vi "_Request Malloc Memory To Factory.vi"(10 "error in (no error)":errorcluster, 11 "CacheSize":i32) -> (2 "error out":errorcluster, 3 "MDPtr DVR":refnum<data-value>)   [LabVIEW 2017, in "MDPtr.lvlib" / "MDPtrMgr.lvclass"]
uses:
  MDPtrMgr.lvclass
  MDPtr TypeDef/MDPtr DataFrame-Memory.ctl
  MDPtr TypeDef/MDPtr DataFrame-Common.ctl
  <vilib>/Utility/Data Type/Type Definitions/Data Type.ctl
  Def-Request.ctl
  Def-Respone.ctl
  MDPtr TypeDef/MDPtr Queue.ctl
  <vilib>/Utility/Data Type/NI_Data Type.lvlib
  MDPtr.lvlib
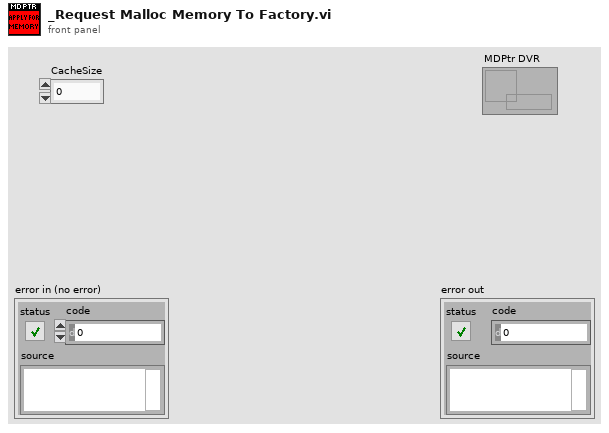
[diagram p1: front panel]
types:
  T1 = typedef "MDPtr.lvlib/MDPtrMgr.lvclass/Def-Respone.ctl" = cluster{"MDPtr DVR":refnum<data-value>, "error out":errorcluster, "MDPtrQueue":T2}
  T2 = typedef "MDPtr.lvlib/MDPtr Queue.ctl" = refnum<queue>
  T3 = typedef "MDPtr.lvlib/MDPtrMgr.lvclass/Def-Request.ctl" = cluster{"Type":enum16{"DVR", "Queue"}, "Cache Length":i32, "ResponeQueue":refnum<queue>}
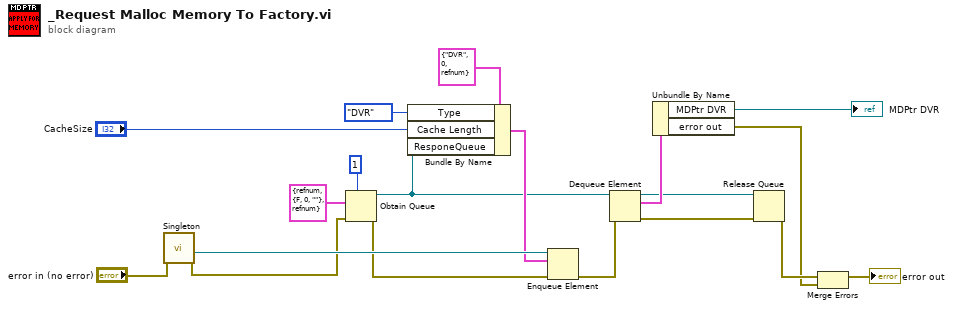
[diagram p0: block diagram]
diagram:
  n1 = call "Singleton.vi"("error in (no error)"="error in (no error)") -> ("error out"=w1:errorcluster, "RequestQueue"=w19:refnum<queue>)  [unwired: 8 in, 1 out]
  n2 = Obtain Queue(max queue size (-1, unlimited)=1, element data type=T1 {"MDPtr DVR"=refnum, "error out"={"status"=FALSE, "code"=0, "source"=""}, "MDPtrQueue"=refnum} ("Request"), error in (no error)=w1) -> (queue out=w11:refnum<queue>, error out=w13:errorcluster)  [unwired: 2 in, 1 out]
  n3 = Bundle By Name(cluster=T3 {"Type"=enum."DVR", "Cache Length"=0, "ResponeQueue"=refnum} ("element"), "Type"=enum16{"DVR", "Queue"}."DVR", "Cache Length"="CacheSize", "ResponeQueue"=w11) -> (w17:T3)
  n4 = Enqueue Element(queue=w19, element=w17, error in (no error)=w13) -> (error out=w10:errorcluster)  [unwired: 1 in, 2 out]
  n5 = Dequeue Element(queue=w11, error in (no error)=w10) -> (queue out=w8:refnum<queue>, element=w9:T1, error out=w6:errorcluster)  [unwired: 1 in, 1 out]
  n6 = Unbundle By Name(w9) -> ("MDPtr DVR"=→"MDPtr DVR":refnum<data-value>, "error out"=w3:errorcluster)
  n7 = Release Queue(queue=w8, error in (no error)=w6) -> (error out=w5:errorcluster)  [unwired: 1 in, 2 out]
  n8 = Merge Errors(w5, w3) -> (→"error out":errorcluster)
